vi "PH_BeamlineInformation.get i attribute.vi"(0 "i ref in":refnum<vi>, 5 "error in (no error)":errorcluster) -> (14 "i ref out":refnum<vi>, 16 "i attribute":T1={"BL GUI Elements of Services"=[], "Powermeters"={"ns FE"={"GUI Ref"=refnum, "Value"=-1.0}, "fs FE"={"GUI Ref"=refnum, "Value"=-1.0}, "PA"={"GUI Ref"=refnum, "Value"=-1.0}, "MA"={"GUI Ref"=refnum, "Value"=-1.0}, "Z6 green"={"GUI Ref"=refnum, "Value"=-1.0}, "Z6 IR"={"GUI Ref"=refnum, "Value"=-1.0}, "Z6 COS"={"GUI Ref"=refnum, "Value"=-1.0}}, "Efficiency"={"PA Gain"={"GUI Ref"=refnum, "Value"=-1.0}, "MA Gain"={"GUI Ref"=refnum, "Value"=-1.0}, "Z6 green Conversion"={"GUI Ref"=refnum, "Value"=-1.0}, "Z6 Comp Losses"={"GUI Ref"=refnum, "Value"=-1.0}}, "Heads"=[]}, 19 "error out":errorcluster)   [LabVIEW 2014, in "PH_BeamlineInformation.lvlib"]
doc: "Gets the i attribute data of an object.\n\nLicense Agreement for this software:\n\nCopyright (C)\nGesellschaft für Schwerionenforschung, GSI\nPlanckstr. 1\n64291 Darmstadt\nGermany\n\nContact: D.Beck@gsi.de \n\nThis program is free software; you can redistribute it and/or modify it under the terms of the GNU General Public License as published by the Free Software Foundation; either version 2 of the license, or (at your option) any later version.\n\nThis program is distributed in the hope that it will be useful, but WITHOUT ANY WARRANTY; without even the implied warranty of MERCHANTABILITY or FITNESS FOR A PARTICULAR PURPOSE. See the GNU General License for more details (http://www.gnu.org).\n\nGesellschaft für Schwerionenforschung, GSI\nPlanckstr. 1, 64291 Darmstadt, Germany\nFor all questions and ideas contact: M.Richter@gsi.de, H.Brand@gsi.de or D.Beck@gsi.de.\nLast update: 17-JUN-2004"
uses:
  PH_BeamlineInformation.lvlib
  PH_BeamlineInformation.i attribute.ctl
  PH_BeamlineInformation.Powermeter.ctl
  PH_BeamlineInformation.Efficiency.ctl
  PH_BeamlineInformation.Head.ctl
  PH_PP_Common/PH_PP_Common.PUs.ctl
  PH_PP_Common/PH_PP_Common.lvlib
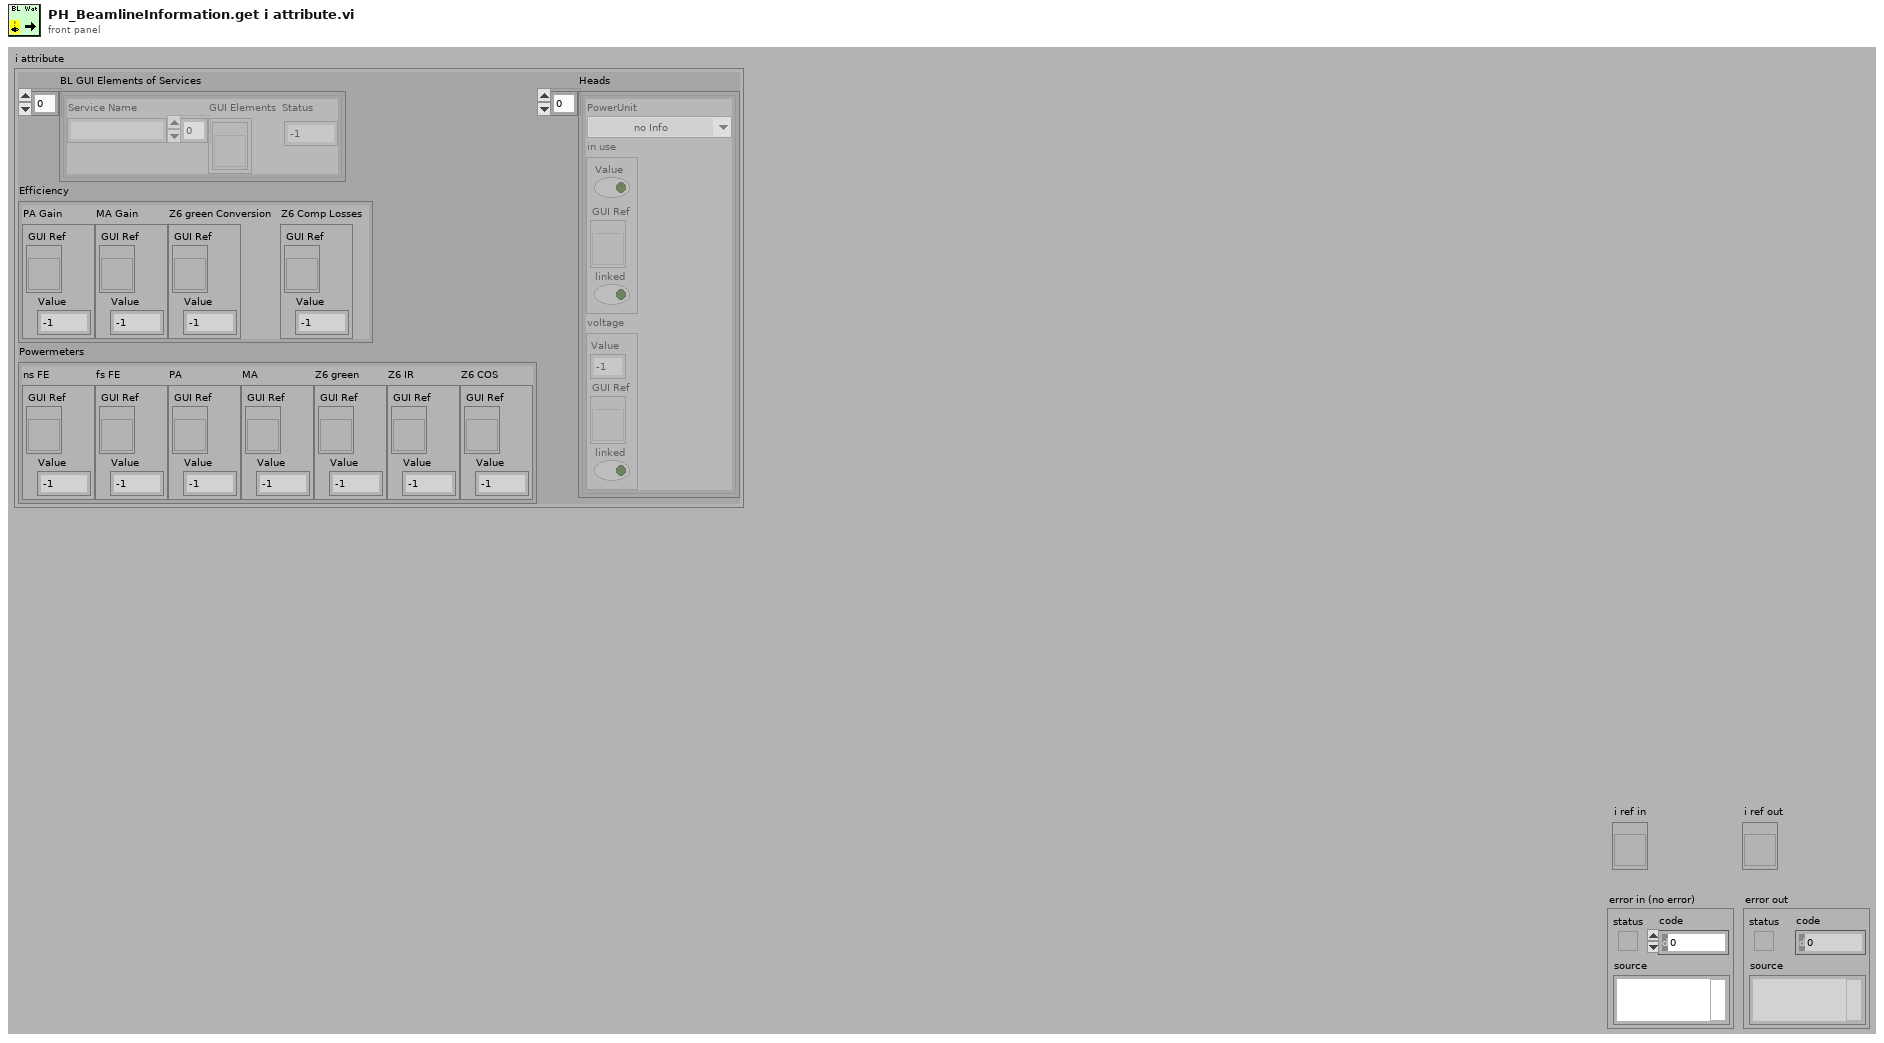
[diagram p1: front panel]
types:
  T1 = typedef "PH_BeamlineInformation.lvlib/PH_BeamlineInformation.i attribute.ctl" = cluster{"BL GUI Elements of Services":cluster{"Service Name":string, "GUI Elements":refnum<vi>[], "Status":i32}[], "Powermeters":T2, "Efficiency":T3, "Heads":T4[]}
  T2 = typedef "PH_BeamlineInformation.lvlib/PH_BeamlineInformation.Powermeter.ctl" = cluster{"ns FE":cluster{"GUI Ref":refnum<vi>, "Value":dbl}, "fs FE":cluster{"GUI Ref":refnum<vi>, "Value":dbl}, "PA":cluster{"GUI Ref":refnum<vi>, "Value":dbl}, "MA":cluster{"GUI Ref":refnum<vi>, "Value":dbl}, "Z6 green":cluster{"GUI Ref":refnum<vi>, "Value":dbl}, "Z6 IR":cluster{"GUI Ref":refnum<vi>, "Value":dbl}, "Z6 COS":cluster{"GUI Ref":refnum<vi>, "Value":dbl}}
  T3 = typedef "PH_BeamlineInformation.lvlib/PH_BeamlineInformation.Efficiency.ctl" = cluster{"PA Gain":cluster{"GUI Ref":refnum<vi>, "Value":dbl}, "MA Gain":cluster{"GUI Ref":refnum<vi>, "Value":dbl}, "Z6 green Conversion":cluster{"GUI Ref":refnum<vi>, "Value":dbl}, "Z6 Comp Losses":cluster{"GUI Ref":refnum<vi>, "Value":dbl}}
  T4 = typedef "PH_BeamlineInformation.lvlib/PH_BeamlineInformation.Head.ctl" = cluster{"PowerUnit":T5, "in use":cluster{"Value":bool, "GUI Ref":refnum<vi>, "linked":bool}, "voltage":cluster{"Value":dbl, "GUI Ref":refnum<vi>, "linked":bool}}
  T5 = typedef "PH_PP_Common.lvlib/PH_PP_Common.PUs.ctl" = enum16{"no Info", "PA-19mm-1", "PA-19mm-2", "PA-45mm-PILC", "PA-45mm-MAIN", "MA-PU-1", "MA-PU-2", "MA-PU-3", "MA-PU-4", "MA-PU-5", "MA-PU-6", "MA-FR", "MA-PILC", "PA-45mm-DP"}
  T6 = enum16{"SetAttribute", "GetAttribute", "CreateAttribute", "DestroyAttribute", "DestroyAllAtributes"}
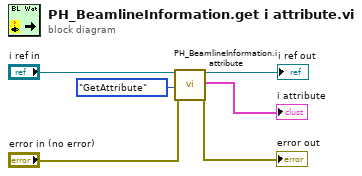
[diagram p0: block diagram]
diagram:
  n1 = call "PH_BeamlineInformation.i attribute.vi"("VI Refnum"="i ref in", "Action"=T6."GetAttribute", "error in (no error)"="error in (no error)") -> ("VI Refnum out"=→"i ref out":refnum<vi>, "CLASS.i attribute out"=→"i attribute":T1, "error out"=→"error out":errorcluster)  [unwired: 14 in]
